vi "Main.vi"() -> ()   [LabVIEW 2020]
doc: "This template is for the Queued Message Handler design pattern.\n\nThe Event Handling Loop generates messages based on user interface actions.\n\nThe Message Handling Loop processes messages generated by the Event Handling Loop, or by other messages. The messages are string values, so new messages can be added easily to the Message Cases case structure in the Message Handling Loop. Each message cluster can also provide an optional value for Message Data, which is a variant that can be converted to whatever message-specific data is required."
uses:
  Controls/UI Data.ctl
  Libraries/Message Queue/Enqueue Message (Single).vi
  <vilib>/Utility/error.llb/Error Cluster From Error Code.vi
  <vilib>/ErrorRing/Error Ring.xnode
  Libraries/Message Queue/Message Queue.lvlib
  Libraries/User Event - Stop/User Event - Stop.lvlib
panel:
  out "Display <Replace Me>":string
  in  "Do Something Else <Replace Me>":bool
  in  "Do Something <Replace Me>":bool
  in  "Exit":bool
  # "These controls have associated \"Value Changed\" events configured in the Event Structure on the diagram.\n\nReplace them (and reconfigure the Event Structure) with the controls you need for your application."
  # "This template is for the Queued Message Handler design pattern.\n\nSee the block diagram for more information on how to use this template."
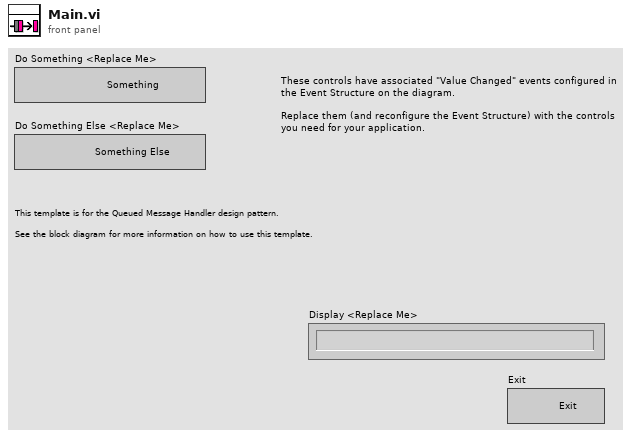
[diagram p1: front panel]
types:
  T1 = typedef "UI Data.ctl" = cluster{"Boolean <Replace Me>":bool, "String <Replace Me>":string, "Numeric <Replace Me>":dbl, "Do Something Ref":refnum<vi>, "Do Something Else Ref":refnum<vi>, "Data Display Ref":refnum<vi>, "Exit Button Ref":refnum<vi>}
  T2 = typedef "Message Queue.lvlib/All Message Queues.ctl" = cluster{"UI":refnum<queue>, "Comm":refnum<queue>, "Data Proecss":refnum<queue>, "File Handling":refnum<queue>}
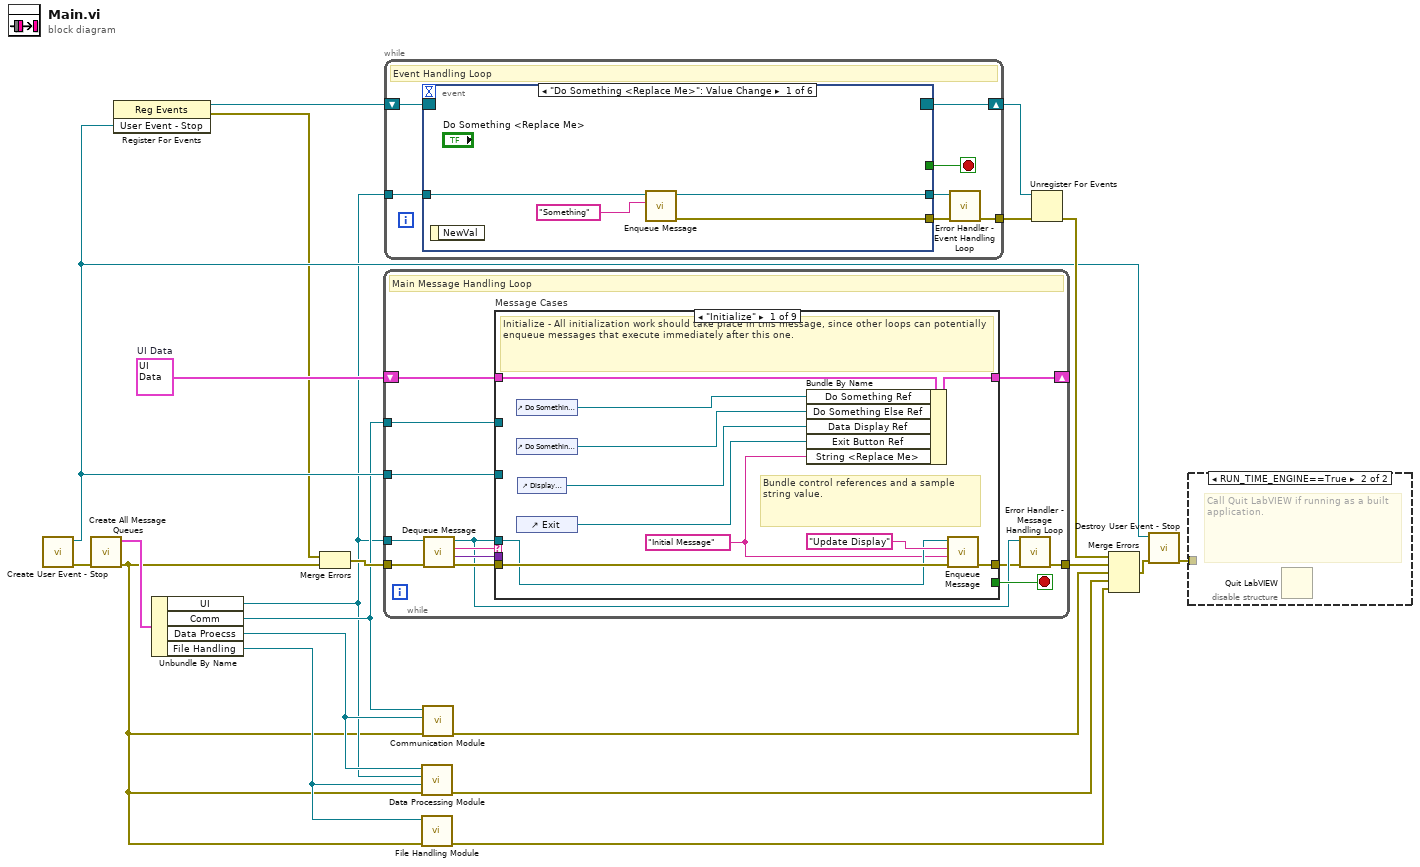
[diagram p0: block diagram]
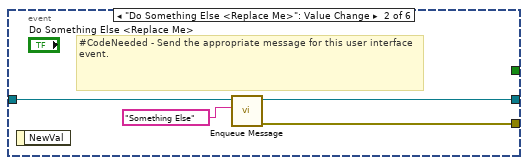
[diagram p3: hidden frame]
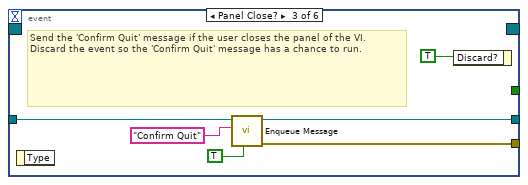
[diagram p4: hidden frame]
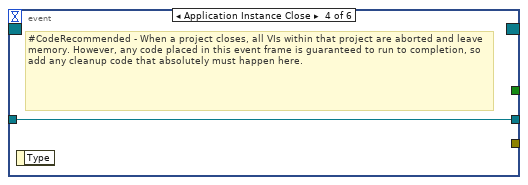
[diagram p5: hidden frame]
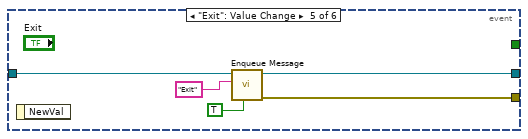
[diagram p6: hidden frame]
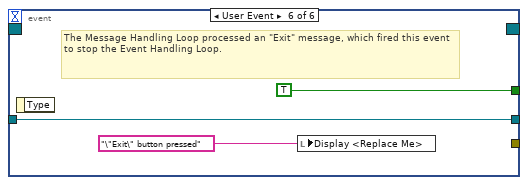
[diagram p7: hidden frame]
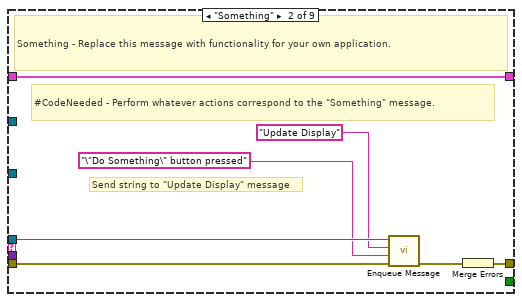
[diagram p8: hidden frame]
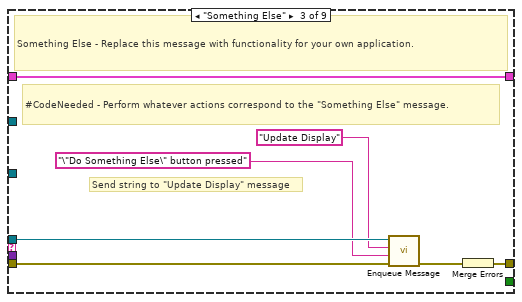
[diagram p9: hidden frame]
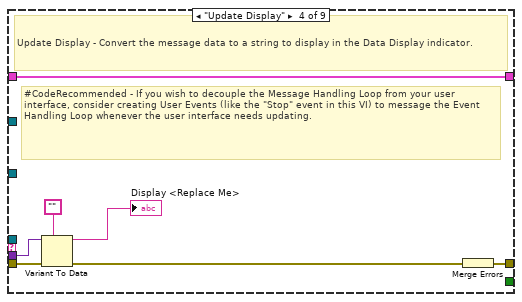
[diagram p10: hidden frame]
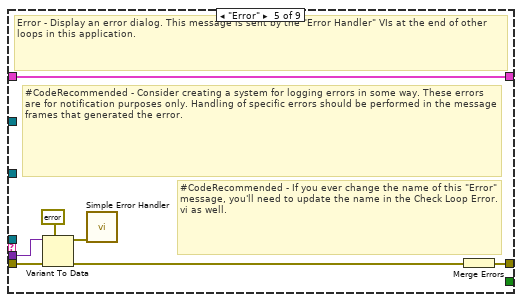
[diagram p11: hidden frame]
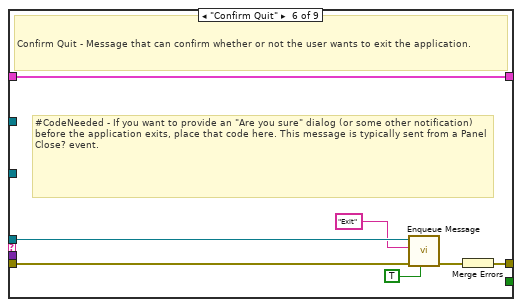
[diagram p12: hidden frame]
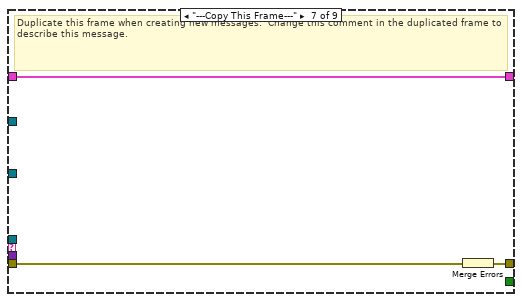
[diagram p13: hidden frame]
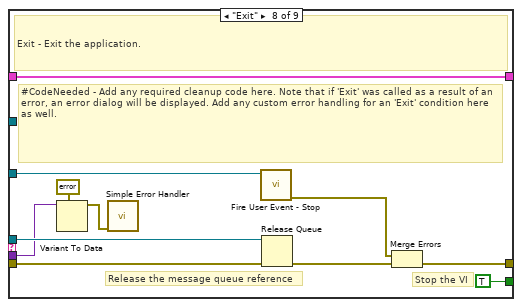
[diagram p14: hidden frame]
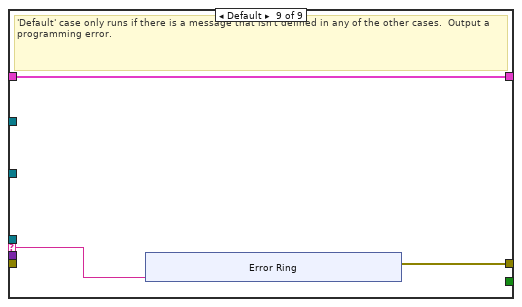
[diagram p15: hidden frame]
diagram:
  w15 = T1 {"Boolean <Replace Me>"=FALSE, "String <Replace Me>"="", "Numeric <Replace Me>"=0.0, "Do Something Ref"=refnum, "Do Something Else Ref"=refnum, "Data Display Ref"=refnum, "Exit Button Ref"=refnum}  # UI Data
  n1 = call "Create User Event - Stop.vi"() -> ("error out"=w19:errorcluster, "User Event - Stop"=w11:refnum<user-event>)  [unwired: 10 in]
  n2 = call "Create All Message Queues.vi"("error in (no error)"=w19) -> ("error out"=w2:errorcluster, "Message Queues out"=w21:T2)  [unwired: 9 in]
  n3 = register-events(w11) -> (reference out=w12:refnum<event-registration>, error out=w9:errorcluster)  [unwired: 2 in]
  n4 = Unbundle By Name(w21) -> ("UI"=w4:refnum<queue>, "Comm"=w7:refnum<queue>, "Data Proecss"=w6:refnum<queue>, "File Handling"=w3:refnum<queue>)
  n5 = Merge Errors(w9, w2) -> (w10:errorcluster)
  n6 = while {
    tunnel: w4 -> [w26]
    shift-right: [w33] -> _
    shift-left: w15 -> [w34]
    tunnel: w11 -> [w31]
    tunnel: w10 -> [w30]
    tunnel: [w24] -> w20
    tunnel: w7 -> [w22]
    stop <- w32 stop-if-true
    # "Main Message Handling Loop"
    n7 = call "Dequeue Message.vi"("error in (no error)"=w30, "Message Queue"=w26) -> ("error out"=w29:errorcluster, "Message Data"=w27:variant, "Message"=w28:string, "dup Message Queue"=w25:refnum<queue>)  [unwired: 6 in]
    n8 = case "Message Cases" shown="\"Initialize\"" w28 {
      selector: w28 -> [_ _ _ _ _ _ _ _ w95]
      tunnel: w25 -> [w36 w48 w55 _ _ w76 _ w94 _]
      tunnel: w29 -> [w44 w50 w57 w64 w73 w80 w83 w87 _]
      tunnel: [w45 w51 w58 w65 w67 w78 w81 w90 w96] -> w23
      tunnel: w34 -> [w43 w52 w59 w66 w72 w79 w82 w93 w97]
      tunnel: [w42 w52 w59 w66 w72 w79 w82 w93 w97] -> w33
      tunnel: [_ _ _ _ _ _ _ TRUE _] -> w32
      tunnel: w27 -> [_ _ _ w63 w71 _ _ w84 _]
      tunnel: w31 -> [_ _ _ _ _ _ _ w89 _]
      tunnel: w22 -> [_ _ _ _ _ _ _ _ _]
      frame "Initialize" {
        w35 = "Initial Message" ("Initial Message")
        # "Bundle control references and a sample string value."
        # "Initialize - All initialization work should take place in this message, since other loops can potentially enqueue messages that execute immediately after this one."
        n9 = control-ref of="Do Something <Replace Me>"() -> (w41:refnum<vi>)
        n10 = control-ref of="Do Something Else <Replace Me>"() -> (w40:refnum<vi>)
        n11 = control-ref of="Exit"() -> (w38:refnum<vi>)
        n12 = control-ref of="Display <Replace Me>"() -> (w39:refnum<vi>)
        n13 = Bundle By Name(cluster=w43, "Do Something Ref"=w41, "Do Something Else Ref"=w40, "Data Display Ref"=w39, "Exit Button Ref"=w38, "String <Replace Me>"=w35) -> (w42:T1)
        n14 = call-poly "Enqueue Message.vi"("error in (no error)"=w44, "Message Data"=w35, "Message"="Update Display", "Message Queue"=w36) -> ("error out"=w45:errorcluster)  [unwired: 6 in, 1 out]
      }
      frame "Something" {
        # "Send string to \"Update Display\" message"
        # "#CodeNeeded - Perform whatever actions correspond to the \"Something\" message."
        # "Something - Replace this message with functionality for your own application."
        n15 = call-poly "Enqueue Message.vi"("error in (no error)"=w50, "Message Data"="\"Do Something\" button pressed" ("\"Do Something\" button pressed"), "Message"="Update Display", "Message Queue"=w48) -> ("error out"=w49:errorcluster)  [unwired: 6 in, 1 out]
        n16 = Merge Errors(w49) -> (w51:errorcluster)
      }
      frame "Something Else" {
        # "Send string to \"Update Display\" message"
        # "#CodeNeeded - Perform whatever actions correspond to the \"Something Else\" message."
        # "Something Else - Replace this message with functionality for your own application."
        n17 = call-poly "Enqueue Message.vi"("error in (no error)"=w57, "Message Data"="\"Do Something Else\" button pressed" ("\"Do Something Else\" button pressed"), "Message"="Update Display", "Message Queue"=w55) -> ("error out"=w56:errorcluster)  [unwired: 6 in, 1 out]
        n18 = Merge Errors(w56) -> (w58:errorcluster)
      }
      frame "Update Display" {
        # "#CodeRecommended - If you wish to decouple the Message Handling Loop from your user interface, consider creating User Events (like the \"Stop\" event in this VI) to message the Event Handling Loop whenever the user interface needs updating."
        # "Update Display - Convert the message data to a string to display in the Data Display indicator."
        n19 = Variant To Data(error in=w64, type="", Variant=w63) -> (data=→"Display <Replace Me>":string, error out=w61:errorcluster)
        n20 = Merge Errors(w61) -> (w65:errorcluster)
      }
      frame "Error" {
        # "#CodeRecommended - If you ever change the name of this \"Error\" message, you'll need to update the name in the Check Loop Error.vi as well."
        # "#CodeRecommended - Consider creating a system for logging errors in some way. These errors are for notification purposes only. Handling of specific errors should be performed in the message frames that generated the error."
        # "Error - Display an error dialog. This message is sent by the \"Error Handler\" VIs at the end of other loops in this application."
        n21 = Variant To Data(error in=w73, type=errorcluster {"status"=FALSE, "code"=0, "source"=""} ("error constant"), Variant=w71) -> (data=w69:errorcluster, error out=w68:errorcluster)
        n22 = call <vilib>:"Simple Error Handler.vi"("error in (no error)"=w69) -> ()  [unwired: 4 in, 5 out]
        n23 = Merge Errors(w68) -> (w67:errorcluster)
      }
      frame "Confirm Quit" {
        # "#CodeNeeded - If you want to provide an \"Are you sure\" dialog (or some other notification) before the application exits, place that code here. This message is typically sent from a Panel Close? event."
        # "Confirm Quit - Message that can confirm whether or not the user wants to exit the application."
        n24 = call-poly "Enqueue Message.vi"("Priority Message? (F)"=TRUE, "error in (no error)"=w80, "Message"="Exit", "Message Queue"=w76) -> ("error out"=w77:errorcluster)  [unwired: 6 in, 1 out]
        n25 = Merge Errors(w77) -> (w78:errorcluster)
      }
      frame "---Copy This Frame---" {
        # "Duplicate this frame when creating new messages.  Change this comment in the duplicated frame to describe this message."
        n26 = Merge Errors(w83) -> (w81:errorcluster)
      }
      frame "Exit" {
        # "Stop the VI"
        # "Release the message queue reference"
        # "#CodeNeeded - Add any required cleanup code here. Note that if 'Exit' was called as a result of an error, an error dialog will be displayed. Add any custom error handling for an 'Exit' condition here as well."
        # "Exit - Exit the application."
        n27 = Variant To Data(type=errorcluster {"status"=FALSE, "code"=0, "source"=""} ("error constant"), Variant=w84) -> (data=w85:errorcluster)  [unwired: 1 in, 1 out]
        n28 = call <vilib>:"Simple Error Handler.vi"("error in (no error)"=w85) -> ()  [unwired: 4 in, 5 out]
        n29 = call "Fire User Event - Stop.vi"("User Event - Stop"=w89) -> ("error out"=w88:errorcluster)  [unwired: 10 in]
        n30 = Release Queue(queue=w94, error in (no error)=w87) -> (error out=w91:errorcluster)  [unwired: 1 in, 2 out]
        n31 = Merge Errors(w88, w91) -> (w90:errorcluster)
      }
      frame Default {
        # "'Default' case only runs if there is a message that isn't defined in any of the other cases.  Output a programming error."
        n32 = xnode "Error Ring"("parameter 0"=w95) -> ("error out"=w96:errorcluster)
      }
    }
    n33 = call "Error Handler - Message Handling Loop.vi"("error in (no error)"=w23, "Message Queue"=w25) -> ("dup error in"=w24:errorcluster)  [unwired: 8 in, 1 out]
  }
  n34 = while {
    tunnel: w4 -> [w111]
    shift-right: [w109] -> w16
    shift-left: w12 -> [w110]
    tunnel: [w105] -> w13
    stop <- w107 stop-if-true
    # "Event Handling Loop"
    n35 = event shown="[0] \"Do Something <Replace Me>\": Value Change" {
      selector: w110 -> [_ _ _ _ _ _]
      dyn-events: [_ _ _ _ _ _] -> w109
      timeout: _ -> [_ _ _ _ _ _]
      tunnel: [_ _ _ _ _ TRUE ("Discard?")] -> w107
      tunnel: w111 -> [w115 w119 w124 w126 w131 w134]
      tunnel: [w112 w116 w123 _ w130 _] -> w108
      tunnel: [w114 w118 w122 w126 w129 w134] -> w106
      event "Do Something <Replace Me>": Value Change {
        n36 = event-data() -> ()  [unwired: 1 in, 1 out]
        n37 = call-poly "Enqueue Message.vi"("Message"="Something", "Message Queue"=w115) -> ("error out"=w112:errorcluster, "dup Message Queue"=w114:refnum<queue>)  [unwired: 8 in]
      }
      event "Do Something Else <Replace Me>": Value Change {
        # "#CodeNeeded - Send the appropriate message for this user interface event."
        n38 = event-data() -> ()  [unwired: 1 in, 1 out]
        n39 = call-poly "Enqueue Message.vi"("Message"="Something Else", "Message Queue"=w119) -> ("error out"=w116:errorcluster, "dup Message Queue"=w118:refnum<queue>)  [unwired: 8 in]
      }
      event Panel Close? {
        # "Send the 'Confirm Quit' message if the user closes the panel of the VI. Discard the event so the 'Confirm Quit' message has a chance to run."
        n40 = event-data() -> ()  [unwired: 1 in, 1 out]
        n41 = call-poly "Enqueue Message.vi"("Priority Message? (F)"=TRUE, "Message"="Confirm Quit", "Message Queue"=w124) -> ("error out"=w123:errorcluster, "dup Message Queue"=w122:refnum<queue>)  [unwired: 7 in]
        n42 = event-data("Discard?"=TRUE) -> ()  [unwired: 1 in, 1 out]
      }
      event Application Instance Close {
        # "#CodeRecommended - When a project closes, all VIs within that project are aborted and leave memory. However, any code placed in this event frame is guaranteed to run to completion, so add any cleanup code that absolutely must happen here."
        n43 = event-data() -> ()  [unwired: 1 in, 1 out]
      }
      event "Exit": Value Change {
        n44 = event-data() -> ()  [unwired: 1 in, 1 out]
        n45 = call-poly "Enqueue Message.vi"("Priority Message? (F)"=TRUE, "Message"="Exit", "Message Queue"=w131) -> ("error out"=w130:errorcluster, "dup Message Queue"=w129:refnum<queue>)  [unwired: 7 in]
      }
      event User Event {
        # "The Message Handling Loop processed an \"Exit\" message, which fired this event to stop the Event Handling Loop."
        n46 = event-data() -> ()  [unwired: 1 in, 1 out]
        n47 = local write "Display <Replace Me>"("\"Exit\" button pressed" ("VI Stopped")) -> ()
      }
    }
    n48 = call "Error Handler - Event Handling Loop.vi"("error in (no error)"=w108, "Message Queue"=w106) -> ("dup error in"=w105:errorcluster)  [unwired: 8 in, 1 out]
  }
  n49 = call "Data Processing Module.vi"("error in (no error)"=w2, "File Handling"=w3, "UI"=w4, "Queue in"=w6) -> ("error out"=w5:errorcluster)  [unwired: 7 in]
  n50 = call "File Handling Module.vi"("error in (no error)"=w2, "Queue in"=w3) -> ("error out"=w1:errorcluster)  [unwired: 9 in]
  n51 = call "Communication Module.vi"("error in (no error)"=w2, "Data Proecss"=w6, "Queue in"=w7) -> ("error out"=w8:errorcluster)  [unwired: 8 in]
  n52 = Unregister For Events(event registration refnum=w16, error in=w13) -> (error out=w17:errorcluster)
  n53 = Merge Errors(w17, w20, w8, w5, w1) -> (w18:errorcluster)
  n54 = call "Destroy User Event - Stop.vi"("error in (no error)"=w18, "User Event - Stop"=w11) -> ("error out"=w14:errorcluster)  [unwired: 9 in]
  n55 = disable-structure shown="RUN_TIME_ENGINE==True" {
    disable-tunnel: w14 -> [_ _]
    frame condition #0 (active) {
    }
    frame condition #1 {
      # "Call Quit LabVIEW if running as a built application."
      n56 = Quit LabVIEW() -> ()  [unwired: 1 in]
    }
  }
